vi "CSUMetClient.vi"() -> (0 "Time Of Value (s)":dbl format="%#.1f", 1 "Error":bool, 2 "RawPressure/mBar":dbl)   [LabVIEW 2011]
panel:
  out "ComputerTime":timestamp
  out "MetTimeStamp":timestamp
  out "data out":string
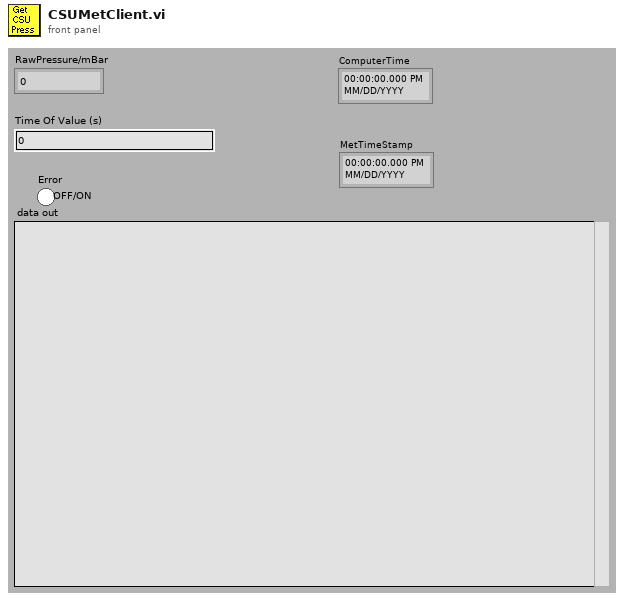
[diagram p1: front panel]
types:
  T1 = cluster{"second":i32, "minute":i32, "hour":i32, "day of month":i32, "month":i32, "year":i32, "day of week":i32, "day of year":i32, "is DST":i32}
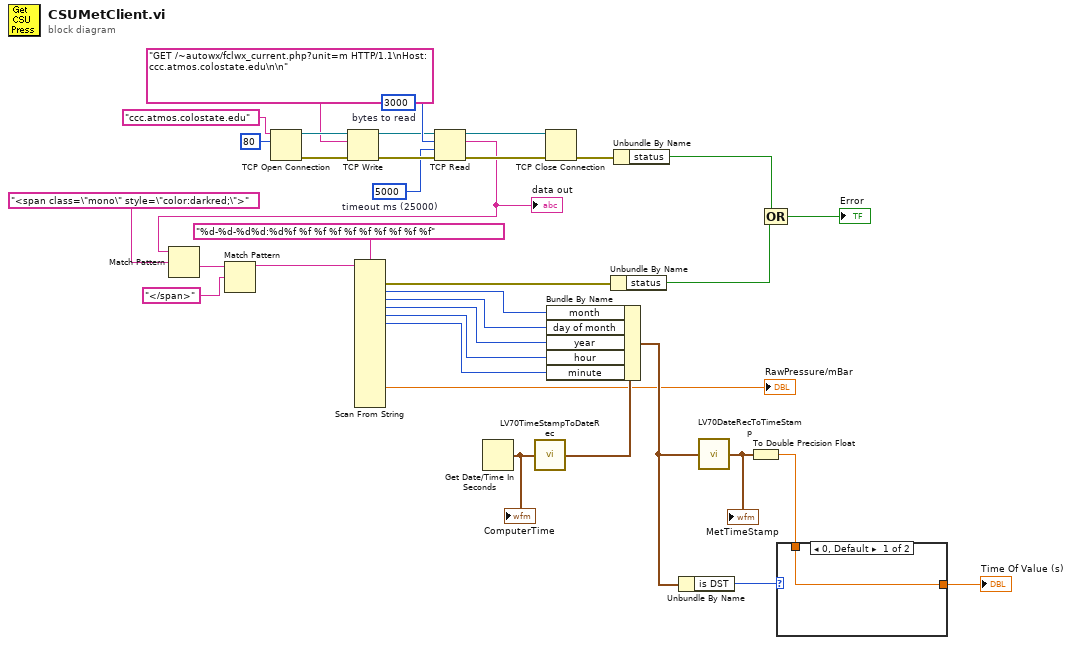
[diagram p0: block diagram]
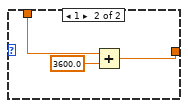
[diagram p2: hidden frame]
diagram:
  w16 = 5000  # timeout ms (25000)
  w27 = 3000  # bytes to read
  n1 = TCP Open Connection(address="ccc.atmos.colostate.edu", remote port or service name=u16 80 ("remote port")) -> (connection ID=w33:refnum<k5>, error out=w31:errorcluster)  [unwired: 1 in, 2 out]
  n2 = TCP Write(connection ID=w33, data in="GET /~autowx/fclwx_current.php?unit=m HTTP/1.1\nHost: ccc.atmos.colostate.edu\n\n", error in (no error)=w31) -> (connection ID out=w26:refnum<k5>, error out=w30:errorcluster)  [unwired: 2 out]
  n3 = TCP Read(connection ID=w26, bytes to read=w27, error in (no error)=w30, 9:w16) -> (connection ID out=w29:refnum<k5>, data out=w11:string, error out=w28:errorcluster)  [unwired: 1 out]
  "data out" <- w11
  n4 = Match Pattern(string=w11, regular expression="<span class=\"mono\" style=\"color:darkred;\">") -> (after substring=w13:string)  [unwired: 4 out]
  n5 = Match Pattern(string=w13, regular expression="</span>") -> (before substring=w10:string)  [unwired: 4 out]
  n6 = Scan From String(format string="%d-%d-%d%d:%d%f %f %f %f %f %f %f %f %f %f", input string=w10) -> (error out=w7:errorcluster, output 1=w2:i32, output 2=w3:i32, output 3=w4:i32, output 4=w5:i32, output 5=w6:i32, output 13=→"RawPressure/mBar":dbl)  [unwired: 2 in, 26 out]
  n7 = Get Date/Time In Seconds() -> (seconds since 1Jan1904=w15:timestamp)
  "ComputerTime" <- w15
  n8 = call <vilib>:"LV70TimeStampToDateRec.vi"("time stamp"=w15) -> ("date time rec"=w25:T1)
  n9 = TCP Close Connection(connection ID=w29, error in (no error)=w28) -> (error out=w20:errorcluster)  [unwired: 2 out]
  n10 = Bundle By Name(cluster=w25, "month"=w2, "day of month"=w3, "year"=w4, "hour"=w5, "minute"=w6) -> (w23:T1)
  n11 = Unbundle By Name(w7) -> ("status"=w8:bool)
  n12 = Unbundle By Name(w20) -> ("status"=w19:bool)
  n13 = Unbundle By Name(w23) -> ("is DST"=w22:i32)
  n14 = call <vilib>:"LV70DateRecToTimeStamp.vi"("date time rec"=w23) -> ("Time Stamp"=w24:timestamp)
  "MetTimeStamp" <- w24
  n15 = To Double Precision Float(number=w24) -> (double precision float=w21:dbl)
  n16 = Compound Arithmetic op=OR(w19, w8) -> (→"Error":bool)
  n17 = case shown="0, Default" w22 {
    tunnel: w21 -> [w36 w39]
    tunnel: [w36 w37] -> w17
    frame 0, Default {
    }
    frame 1 {
      n18 = Add(x=w39, y=3600.0) -> (x+y=w37:dbl)
    }
  }
  "Time Of Value (s)" <- w17
